vi "SetTimer FGV.vi"(1 "Logging Rate":T1) -> (0 "Add?":bool=TRUE)   [LabVIEW 2018]
uses:
  Ctls/LoggingRate.ctl
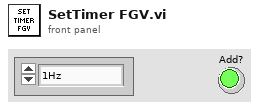
[diagram p1: front panel]
types:
  T1 = typedef "LoggingRate.ctl" = enum16{"1Hz", "2Hz", "5Hz", "10Hz"}
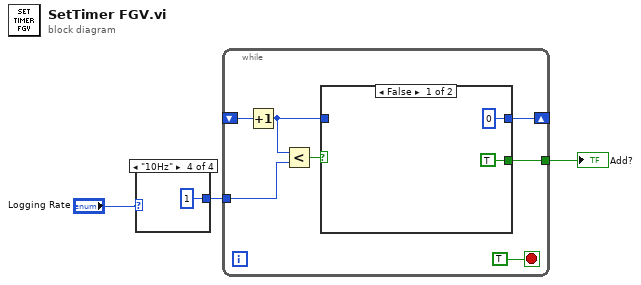
[diagram p0: block diagram]
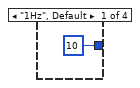
[diagram p2: hidden frame]
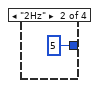
[diagram p3: hidden frame]
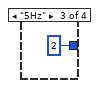
[diagram p4: hidden frame]
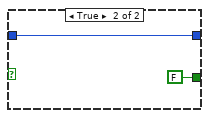
[diagram p5: hidden frame]
diagram:
  n1 = case shown="\"10Hz\"" "Logging Rate" {
    tunnel: [u16 10 u16 5 u16 2 u16 1] -> w1
    frame "1Hz", Default {
    }
    frame "2Hz" {
    }
    frame "5Hz" {
    }
    frame "10Hz" {
    }
  }
  n2 = while {
    shift-right: [w12] -> _
    shift-left: _ -> [w10]
    tunnel: [w11] -> w3
    tunnel: w1 -> [w8]
    stop <- TRUE stop-if-true
    n3 = Increment(x=w10) -> (x+1=w9:u8)
    n4 = Less?(x=w9, y=w8) -> (x < y?=w13:bool)
    n5 = case shown="False" w13 {
      tunnel: w9 -> [_ w17]
      tunnel: [u8 0 w17] -> w12
      tunnel: [TRUE FALSE] -> w11
      frame False {
      }
      frame True {
      }
    }
  }
  "Add?" <- w3
